vi "RT Driver VI.vi"(7 "Operation":T1, 11 "Device Reference in":T2 format="%.0x") -> (0 "Error Code":i32)   [LabVIEW 2020, in "Communication Bus Template Engine.lvlib" / "Custom Device.lvlib"]
uses:
  Custom Device.lvlib
  <vilib>/NI VeriStand/Custom Device API/Custom Device Item Ref.ctl
  <vilib>/NI VeriStand/Custom Device API/Hardware Interface Driver VI Operation.ctl
  Compiled.Settings.ctl
  Inline Execution Unit Compiled Information.ctl
  <vilib>/NI VeriStand/Custom Device API/Data Reference.ctl
  <vilib>/NI VeriStand/Custom Device API/Block Data Reference.ctl
  Asynchronous Execution Unit Compiled Information.ctl
  RTStateVariables.ctl
  <vilib>/NI/NIVS Inline Async API/_VS Inline Async API/VS Inline Async API/VS Inline Async API.lvclass
  Inline Execution Unit Runtime Information.ctl
  Interfaces/Execution Unit/Execution Unit.lvclass
  Asynchronous Execution Unit Runtime Information.ctl
  Interfaces/Shared Resources/Shared Resources.lvclass
  <vilib>/NI/NIVS Inline Async API/_VS Inline Async API/VS Inline Async API/VS Inline Async API.lvclass/VS Inline Async API.ctl
  <vilib>/NI/NIVS Inline Async API/_Data Access Engine/Data Access Engine/Data Access Engine.lvclass/Data Access Engine.ctl
  <vilib>/NI/NIVS Inline Async API/_Data Access Engine/Access Type Classes/Write/Write.lvclass/Write.ctl
  <vilib>/NI/NIVS Inline Async API/_Data Access Engine/Access Type Classes/ReadWrite/ReadWrite.lvclass/ReadWrite.ctl
  <vilib>/NI/NIVS Inline Async API/_Data Access Engine/Access Type Classes/Read/Read.lvclass/Read.ctl
  <vilib>/NI/NIVS Inline Async API/_Data Access Engine/Data Access Engine/Methods/Data.Engine.Read Data from HW.vi
  <vilib>/NI/NIVS Inline Async API/_VS Inline Async API/Error Handling Process/SubVIs/Error.GetError.vi
  <vilib>/NI/NIVS Inline Async API/_Data Access Engine/Data Access Engine/Methods/Data.Engine.Write Data to HW.vi
  <vilib>/NI/NIVS Inline Async API/_Data Access Engine/Access Type Classes/ReadWrite/ReadWrite.EngineData.vi
  <vilib>/NI/NIVS Inline Async API/_Data Access Engine/Access Type Classes/Write/Write.EngineData.vi
  <vilib>/NI/NIVS Inline Async API/_Data Access Engine/Access Type Classes/Read/Read.EngineData.vi
  <vilib>/NI VeriStand/Custom Device API/NI VeriStand - Get Channel Value by Data Reference.vi
  <vilib>/NI VeriStand/Custom Device API/NI VeriStand - Set Channel Value by Data Reference.vi
  <vilib>/NI VeriStand/Custom Device API/NI VeriStand - Get Channel Values by Block Data Reference.vi
  Scripting/Constants.vi
  <vilib>/NI VeriStand/Custom Device API/Get Item Property (Variant).vi
  <vilib>/NI VeriStand/Custom Device API/Global Data Refs.vi
  <vilib>/NI VeriStand/Custom Device API/Custom Device API.lvlib
  <vilib>/NI VeriStand/Custom Device Tools/Custom Device Utility Library/Custom Device Utility Library.lvlib
  Scripting/Communication Bus Template Scripting.lvlib
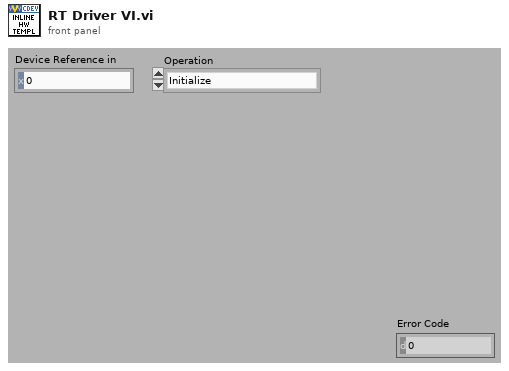
[diagram p1: front panel]
types:
  T1 = typedef "Custom Device API.lvlib/Hardware Interface Driver VI Operation.ctl" = enum16{"Initialize", "Start", "Read Data from HW", "Write Data to HW", "Close"}
  T2 = typedef "Custom Device API.lvlib/Custom Device Item Ref.ctl" = u64
  T3 = typedef "Communication Bus Template Engine.lvlib/Custom Device.lvlib/RTStateVariables.ctl" = cluster{"Async":refnum<class "VS Inline Async API.lvclass">, "Inline Execution Units":T4[], "Asynchronous Execution Units":T7[], "shared resources":refnum<class "Shared Resources.lvclass">}
  T4 = typedef "Communication Bus Template Engine.lvlib/Custom Device.lvlib/Inline Execution Unit Runtime Information.ctl" = cluster{"Execution Unit":refnum<class "Execution Unit.lvclass">, "Incoming Buffer":dbl[], "Outgoing Buffer":dbl[], "Incoming Data References":T5[], "Outgoing Data References":T6[]}
  T5 = typedef "Custom Device API.lvlib/Data Reference.ctl" = i32
  T6 = typedef "Custom Device API.lvlib/Block Data Reference.ctl" = cluster{"Data Reference":T5, "Offset":u64, "Length":u64}
  T7 = typedef "Communication Bus Template Engine.lvlib/Custom Device.lvlib/Asynchronous Execution Unit Runtime Information.ctl" = cluster{"Execution Unit":refnum<class "Execution Unit.lvclass">, "Incoming Channel Group Name":string, "Outgoing Channel Group Name":string, "ReadWrite Channel Group Name":string}
  T8 = typedef "Communication Bus Template Engine.lvlib/Custom Device.lvlib/Compiled.Settings.ctl" = cluster{"Name":string, "Inline Execution Unit Compiled Information":T9[], "Asynchronous Execution Unit Compiled Information":T10[], "Flattened Shared Resources":string}
  T9 = typedef "Communication Bus Template Engine.lvlib/Custom Device.lvlib/Inline Execution Unit Compiled Information.ctl" = cluster{"Flattened Execution Unit":string, "Incoming Buffer":dbl[], "Outgoing Buffer":dbl[], "Incoming Data References":T5[], "Outgoing Data References":T6[]}
  T10 = typedef "Communication Bus Template Engine.lvlib/Custom Device.lvlib/Asynchronous Execution Unit Compiled Information.ctl" = cluster{"Flattened Execution Unit":string, "Incoming Channel Group Name":string, "Outgoing Channel Group Name":string, "ReadWrite Channel Group Name":string}
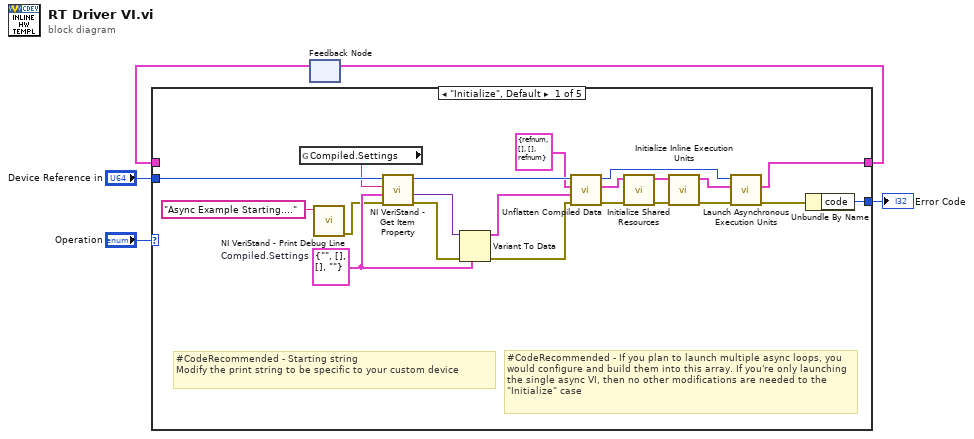
[diagram p0: block diagram]
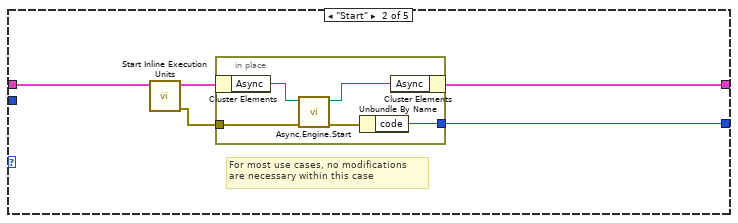
[diagram p2: hidden frame]
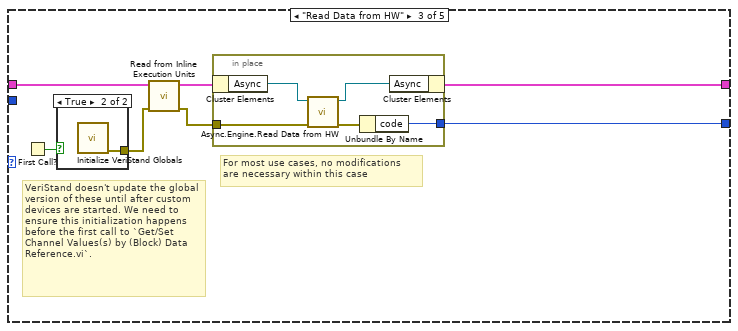
[diagram p3: hidden frame]
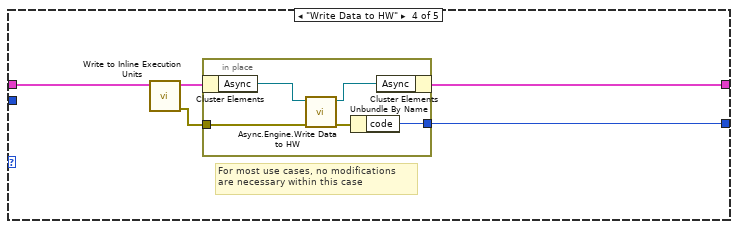
[diagram p5: hidden frame]
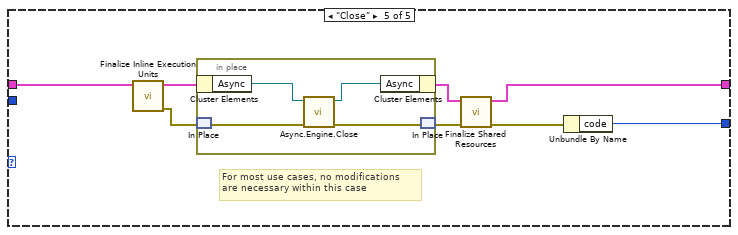
[diagram p6: hidden frame]
diagram:
  n1 = feedback #1() -> (w3:T3)  [unwired: 1 out]
  n2 = case shown="\"Initialize\", Default" "Operation" {
    tunnel: [w12 w30 w42 w53 w61] -> w4
    tunnel: w3 -> [_ w31 w41 w52 w67]
    tunnel: "Device Reference in" -> [w25 _ _ _ _]
    tunnel: [w26 w29 w43 w54 w64] -> w1
    frame "Initialize", Default {
      w21 = T8 {"Name"="", "Inline Execution Unit Compiled Information"=[], "Asynchronous Execution Unit Compiled Information"=[], "Flattened Shared Resources"=""}  # Compiled.Settings
      # "#CodeRecommended - Starting string\nModify the print string to be specific to your custom device"
      # "#CodeRecommended - If you plan to launch multiple async loops, you would configure and build them into this array. If you're only launching the single async VI, then no other modifications are needed to the \"Initialize\" case"
      n3 = global read "Constants.vi" "Compiled.Settings"() -> (w22:string)
      n4 = call <vilib>:"NI VeriStand - Print Debug Line.vi"("Message"="Async Example Starting....") -> ("error out"=w20:errorcluster)  [unwired: 10 in]
      n5 = call-poly <vilib>:"NI VeriStand - Get Item Property.vi"("error in (no error)"=w20, "Default Value"=w21, "Property Name"=w22, "Item Ref in"=w25) -> ("error out"=w24:errorcluster, "Value"=w23:variant, "Item Ref out"=w15:T2)  [unwired: 4 in, 1 out]
      n6 = Variant To Data(error in=w24, type=w21, Variant=w23) -> (data=w17:T8, error out=w16:errorcluster)
      n7 = call "Unflatten Compiled Data.vi"("error in (no error)"=w16, "Compiled.Settings"=w17, "RTStateVariables in"=T3 {"Async"=refnum, "Inline Execution Units"=[], "Asynchronous Execution Units"=[], "shared resources"=refnum} ("RTStateVariables"), "Item Ref in"=w15) -> ("error out"=w9:errorcluster, "RTStateVariables out"=w6:T3, "Item Ref out"=w11:T2)  [unwired: 5 in]
      n8 = call "Initialize Shared Resources.vi"("error in"=w9, "RTStateVariables in"=w6) -> ("error out"=w8:errorcluster, "RTStateVariables out"=w7:T3)  [unwired: 8 in]
      n9 = call "Initialize Inline Execution Units.vi"("error in"=w8, "RTStateVariables in"=w7) -> ("error out"=w13:errorcluster, "RTStateVariables out"=w10:T3)  [unwired: 8 in]
      n10 = call "Launch Asynchronous Execution Units.vi"("error in (no error)"=w13, "RTStateVariables in"=w10, "Device Ref in"=w11) -> ("error out"=w18:errorcluster, "RTStateVariables out"=w12:T3)  [unwired: 6 in, 1 out]
      n11 = Unbundle By Name(w18) -> ("code"=w26:i32)
    }
    frame "Start" {
      # "For most use cases, no modifications \nare necessary within this case"
      n12 = call "Start Inline Execution Units.vi"("RTStateVariables in"=w31) -> ("error out"=w27:errorcluster, "RTStateVariables out"=w28:T3)  [unwired: 9 in]
      n13 = in-place {
        in-place-border: [w33] -> w29
        in-place-border: w27 -> [w32]
        n14 = in-place-cluster #2(w28) -> ("Async"=w36:refnum<class "VS Inline Async API.lvclass">)
        n15 = call <vilib>:"Async.Engine.Start.vi"("error in (no error)"=w32, "VS Inline Async API in"=w36) -> ("error out"=w34:errorcluster, "VS Inline Async API out"=w35:refnum<class "VS Inline Async API.lvclass">)  [unwired: 8 in]
        n16 = Unbundle By Name(w34) -> ("code"=w33:i32)
        n17 = in-place-cluster #2("Async"=w35) -> (w30:T3)
      }
    }
    frame "Read Data from HW" {
      # "VeriStand doesn't update the global version of these until after custom devices are started. We need to ensure this initialization happens before the first call to `Get/Set Channel Values(s) by (Block) Data Reference.vi`."
      # "For most use cases, no modifications \nare necessary within this case"
      n18 = First Call?() -> (First Call?: T/F=w38:bool)
      n19 = case shown="True" w38 {
        tunnel: [_ w44] -> w37
        frame False {
        }
        frame True {
          n20 = call "Initialize VeriStand Globals.vi"() -> ("error out"=w44:errorcluster)  [unwired: 11 in]
        }
      }
      n21 = call "Read from Inline Execution Units.vi"("error in (no error)"=w37, "RTStateVariables in"=w41) -> ("error out"=w39:errorcluster, "RTStateVariables out"=w40:T3)  [unwired: 8 in]
      n22 = in-place {
        in-place-border: [w47] -> w43
        in-place-border: w39 -> [w45]
        n23 = in-place-cluster #3(w40) -> ("Async"=w49:refnum<class "VS Inline Async API.lvclass">)
        n24 = call <vilib>:"Async.Engine.Read Data from HW.vi"("error in"=w45, "Async in"=w49) -> ("error out"=w46:errorcluster, "Async out"=w48:refnum<class "VS Inline Async API.lvclass">)  [unwired: 8 in]
        n25 = Unbundle By Name(w46) -> ("code"=w47:i32)
        n26 = in-place-cluster #3("Async"=w48) -> (w42:T3)
      }
    }
    frame "Write Data to HW" {
      # "For most use cases, no modifications \nare necessary within this case"
      n27 = call "Write to Inline Execution Units.vi"("RTStateVariables in"=w52) -> ("error out"=w50:errorcluster, "RTStateVariables out"=w51:T3)  [unwired: 9 in]
      n28 = in-place {
        in-place-border: [w59] -> w54
        in-place-border: w50 -> [w55]
        n29 = in-place-cluster #4(w51) -> ("Async"=w57:refnum<class "VS Inline Async API.lvclass">)
        n30 = call <vilib>:"Async.Engine.Write Data to HW.vi"("error in (no error)"=w55, "VS Inline Async API in"=w57) -> ("error out"=w58:errorcluster, "VS Inline Async API out"=w56:refnum<class "VS Inline Async API.lvclass">)  [unwired: 8 in]
        n31 = Unbundle By Name(w58) -> ("code"=w59:i32)
        n32 = in-place-cluster #4("Async"=w56) -> (w53:T3)
      }
    }
    frame "Close" {
      # "For most use cases, no modifications \nare necessary within this case"
      n33 = call "Finalize Inline Execution Units.vi"("RTStateVariables in"=w67) -> ("error out"=w65:errorcluster, "RTStateVariables out"=w66:T3)  [unwired: 9 in]
      n34 = in-place {
        n35 = in-place-cluster #5(w66) -> ("Async"=w71:refnum<class "VS Inline Async API.lvclass">)
        n36 = in-place-match #6(w65) -> (w69:errorcluster)
        n37 = call <vilib>:"Async.Engine.Close.vi"("error in (no error)"=w69, "Async in"=w71) -> ("error out"=w68:errorcluster, "Async out"=w70:refnum<class "VS Inline Async API.lvclass">)  [unwired: 8 in]
        n38 = in-place-cluster #5("Async"=w70) -> (w62:T3)
        n39 = in-place-match #6(w68) -> (w63:errorcluster)
      }
      n40 = call "Finalize Shared Resources.vi"("error in"=w63, "RTStateVariables in"=w62) -> ("error out"=w60:errorcluster, "RTStateVariables out"=w61:T3)  [unwired: 8 in]
      n41 = Unbundle By Name(w60) -> ("code"=w64:i32)
    }
  }
  "Error Code" <- w1
  n42 = feedback-in #1(w4) -> ()
